vi "APC_9056_NI9205conf.vi"() -> (0 "Min V out":dbl[](array[numeric])=[-10.0, -10.0, -10.0, -10.0, -10.0, -10.0, -10.0, -10.0, -10.0, -10.0, -10.0, -10.0, -10.0, -10.0, -10.0, -10.0], 1 "Max V out":dbl[](array[numeric])=[10.0, 10.0, 10.0, 10.0, 10.0, 10.0, 10.0, 10.0, 10.0, 10.0, 10.0, 10.0, 10.0, 10.0, 10.0, 10.0], 2 "scaled units out2":string[](array[string])=["bar", "perc", "perc", "r", "perc", "r", "ppm", "bar", "Nm", "V", "V", "V", "V", "V", "V", "V"], 3 "Y-Intercept out":dbl[](array[numeric]) format="%.2g", 4 "Slope out":dbl[](array[numeric])=[1.0, 1.0, 1.0, 1.0, 1.0, 1.0, 1.0, 1.0, 1.0, 1.0, 1.0, 1.0, 1.0, 1.0, 1.0, 1.0] format="%.2g", 5 "channels name out":string[](array[string])=["WF-PT-001_bar", "WF-OA-001-O2_perc", "WF-OA-001-O2corr_perc", "WF-OA-001-Lambda_r", "WF-OA-002-O2_perc", "WF-OA-002-Lambda_r", "WF-OA-002-NOx_ppm", "EO-PT-001_bar", "TORQUE_Nm", "NI9205_9_V", "NI9205_10_V", "NI9205_11_V", "NI9205_12_V", "NI9205_13_V", "NI9205_14_V", "NI9205_15_V"])   [LabVIEW 2020]
panel:
  in  "Min V":dbl[](array[numeric])=[-10.0, -10.0, -10.0, -10.0, -10.0, -10.0, -10.0, -10.0, -10.0, -10.0, -10.0, -10.0, -10.0, -10.0, -10.0, -10.0]
  in  "Max V":dbl[](array[numeric])=[10.0, 10.0, 10.0, 10.0, 10.0, 10.0, 10.0, 10.0, 10.0, 10.0, 10.0, 10.0, 10.0, 10.0, 10.0, 10.0]
  in  "scaled units":string[](array[string])=["bar", "perc", "perc", "r", "perc", "r", "ppm", "bar", "Nm", "V", "V", "V", "V", "V", "V", "V"]
  in  "Y-Intercept":dbl[](array[numeric])=[0.0, 0.0, 0.0, 0.0, 0.0, 0.0, 0.0, 0.0, 0.0, 0.0, 0.0, 0.0, 0.0, 0.0, 0.0, 0.0] format="%.2g"
  in  "Slope":dbl[](array[numeric])=[1.0, 1.0, 1.0, 1.0, 1.0, 1.0, 1.0, 1.0, 1.0, 1.0, 1.0, 1.0, 1.0, 1.0, 1.0, 1.0] format="%.2g"
  in  "channels name":string[](array[string])=["WF-PT-001", "WF-OA-001-O2", "WF-OA-001-O2corr", "WF-OA-001-Lambda", "WF-OA-002-O2", "WF-OA-002-Lambda", "WF-OA-002-NOx", "EO-PT-001", "TORQUE", "NI9205_9", "NI9205_10", "NI9205_11", "NI9205_12", "NI9205_13", "NI9205_14", "NI9205_15"]
  # "NI9205"
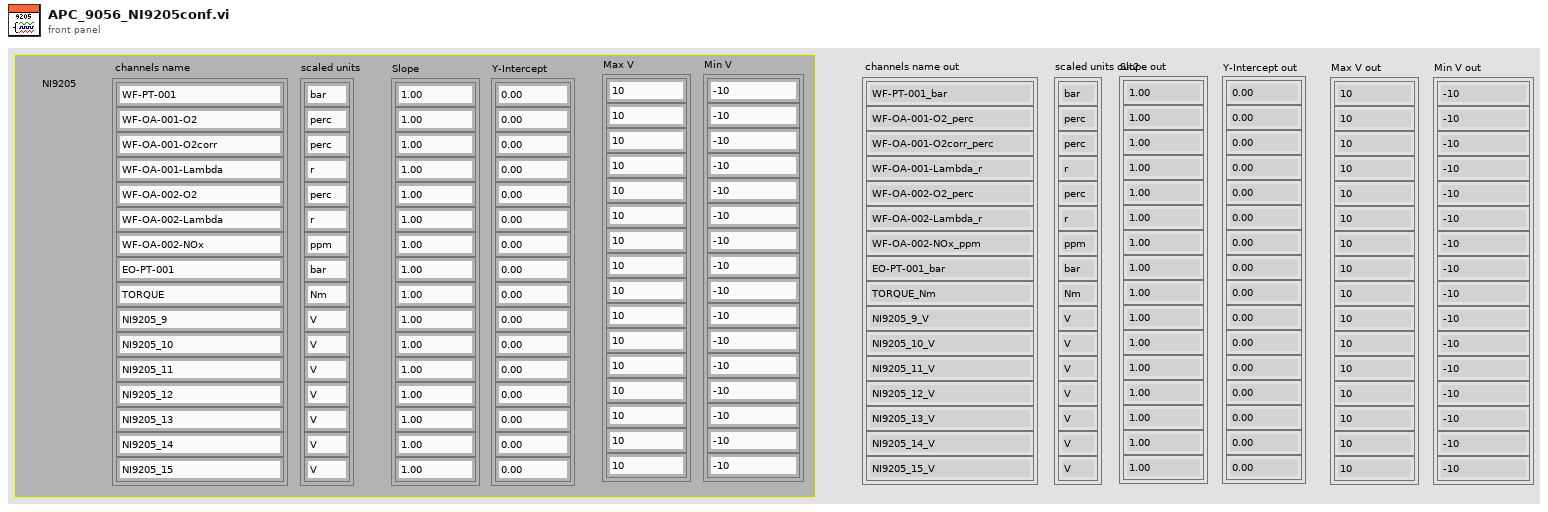
[diagram p1: front panel]
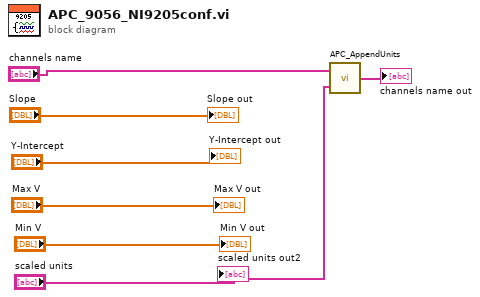
[diagram p0: block diagram]
diagram:
  n1 = call "APC_AppendUnits.vi"("units"="scaled units", "names"="channels name") -> ("names_units"=→"channels name out":string[])
  "Slope out" <- "Slope"
  "Y-Intercept out" <- "Y-Intercept"
  "Max V out" <- "Max V"
  "Min V out" <- "Min V"
  "scaled units out2" <- "scaled units"
